vi "Vor Lin Check Benutzerabfrage.vi"() -> ()   [LabVIEW 2020, in "Linearisierung v2.lvlib" / "Gasteiler.lvlib"]
uses:
  Gasteiler.lvlib
  AK-Komm Gasteiler/Aktionen AK Komm.ctl
  AK-Komm Gasteiler/AK Komm Gasteiler.lvlib
  Lin Daten verwalten Aktionen.ctl
  Stufen Tabelle.ctl
  Aktionen FGV Gasteiler Daten.ctl
  AK-Komm Gasteiler/Alter Gasteiler/Aktionen AK Komm_ALT.ctl
  AK-Komm Gasteiler/Alter Gasteiler/Alter Gasteiler.lvlib
  Allgemein/allgemeine Sub-VIs.lvlib
  Sprachverwaltung/Sprachverwaltung.lvlib
  Visualisierungs Elemente/Zahlen-Eingabefeld.ctl
  Horiba/Horiba GDC.lvlib
  Horiba/Aktion Befehl.ctl
  Sprachverwaltung/FGV Aktion Tabelle zerlegen.ctl
  Visualisierungs Elemente/Button.ctl
panel:
  in  "Stufen Tabelle 2":T1
  in  "Abbrechen":T2
  in  "OK":T2
  out "Stufen Tabelle":T1
  out "AGAK":string[](array[string])
  # "Parameter Kontrolle"
  # "Inlet Gas:"
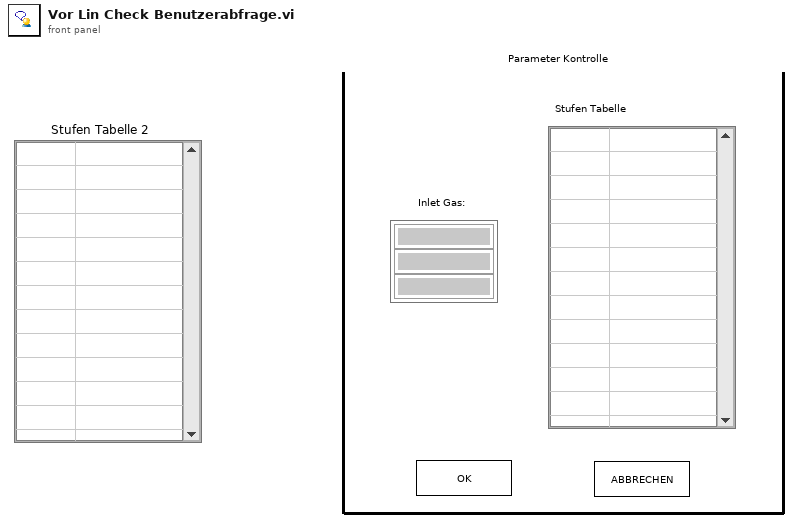
[diagram p1: front panel]
types:
  T1 = typedef "Linearisierung v2.lvlib/Gasteiler.lvlib/Stufen Tabelle.ctl" = string[][]
  T2 = typedef "Button.ctl" = bool
  T3 = typedef "Sprachverwaltung.lvlib/FGV Aktion Tabelle zerlegen.ctl" = enum16{"laden", "vereinzeln", "speichern"}
  T4 = enum8{"Enabled", "Disabled", "Disabled and Grayed Out"}
  T5 = typedef "Linearisierung v2.lvlib/Gasteiler.lvlib/Aktionen FGV Gasteiler Daten.ctl" = enum16{"lesen", "Gasteiler Daten", "Seriellen Param.", "MB-Endwert", "laden", "speichern", "Anforderung", "TCP", "Aufzeichnung Start"}
  T6 = typedef "Linearisierung v2.lvlib/Gasteiler.lvlib/Lin Daten verwalten Aktionen.ctl" = enum16{"lesen", "speichern", "laden", "Lin Daten schr.", "Stufen Tabelle", "Lin Name AK", "Lin Pfad AK", "Umkehren"}
  T7 = typedef "Linearisierung v2.lvlib/Gasteiler.lvlib/AK Komm Gasteiler.lvlib/Aktionen AK Komm.ctl" = enum16{"lesen", "initialisieren", "beenden", "Status", "SMAN", "SREM", "STBY", "ASTF", "ASTZ", "SLST", "AGAT", "EGAK", "AGAK", "AKAK", "ADRU", "SKOP", "SVSA", "SVSZ", "SONO", "SAIR", "SNOX", "ANOX", "SSPL", "SRUC", "SLIN", "ALST", "ETYP", "SVIO", "LCYL", "CCYL", "DCYL", "SCYL", "GCYL", "DRGV", "DRDC"}
  T8 = typedef "Linearisierung v2.lvlib/Gasteiler.lvlib/AK Komm Gasteiler.lvlib/Alter Gasteiler.lvlib/Aktionen AK Komm_ALT.ctl" = enum16{"lesen", "initialisieren", "beenden", "SRES", "STBY", "SREM", "SMAN", "SLIN", "SLCH", "SLST", "SSPL", "AGAT", "ALST", "ASTZ", "ASTF", "AGAK", "EGAK"}
  T9 = typedef "Linearisierung v2.lvlib/Gasteiler.lvlib/Horiba GDC.lvlib/Aktion Befehl.ctl" = enum16{"lesen", "initialisieren", "Beenden", "Standby", "GD/CC", "Info", "Flow", "Alarm", "GD parameter", "GD point", "Durchfluss", "Spuelen1", "Spuelen1 On", "Spuelen1Off", "Spuelen2", "Ventil-Abfrage", "Reset"}
  T10 = typedef "Zahlen-Eingabefeld.ctl" = sgl
  T11 = typedef "Linearisierung v2.lvlib/Gasteiler.lvlib/Gasteiler Daten.ctl" = cluster{"Gasteiler":T12, "Gasteiler Stufen":T13, "Gasteiler Type":T14, "Konfig Gasteiler":T15, "Gasteiler Span Eingänge":u16}
  T12 = typedef "String - Eingabefeld.ctl" = string
  T13 = typedef "Linearisierung v2.lvlib/Gasteiler.lvlib/Gasteiler Stufen.ctl" = u16
  T14 = typedef "Linearisierung v2.lvlib/GasteilerType.ctl" = u16
  T15 = typedef "System Einstellungen V2.lvlib/Gasteiler Auswahl.ctl" = u16
  T16 = typedef "Linearisierung v2.lvlib/Gasteiler.lvlib/Lin Daten.ctl" = cluster{"PrüfgasName":T12, "Verdünnungsgas":T17, "Anzahl Stufen":T10, "Zeitdauer Stufe":T10, "Max Fehler (Sollwert)":T10, "Bearbeiter":T12, "Kalibriergerät":T12, "Mittelwerte":i32, "Komponente":u16, "CalGas Eingang":u16, "Konzentration":sgl}
  T17 = typedef "Linearisierung v2.lvlib/Gasteiler.lvlib/Prüfgas in.ctl" = u16
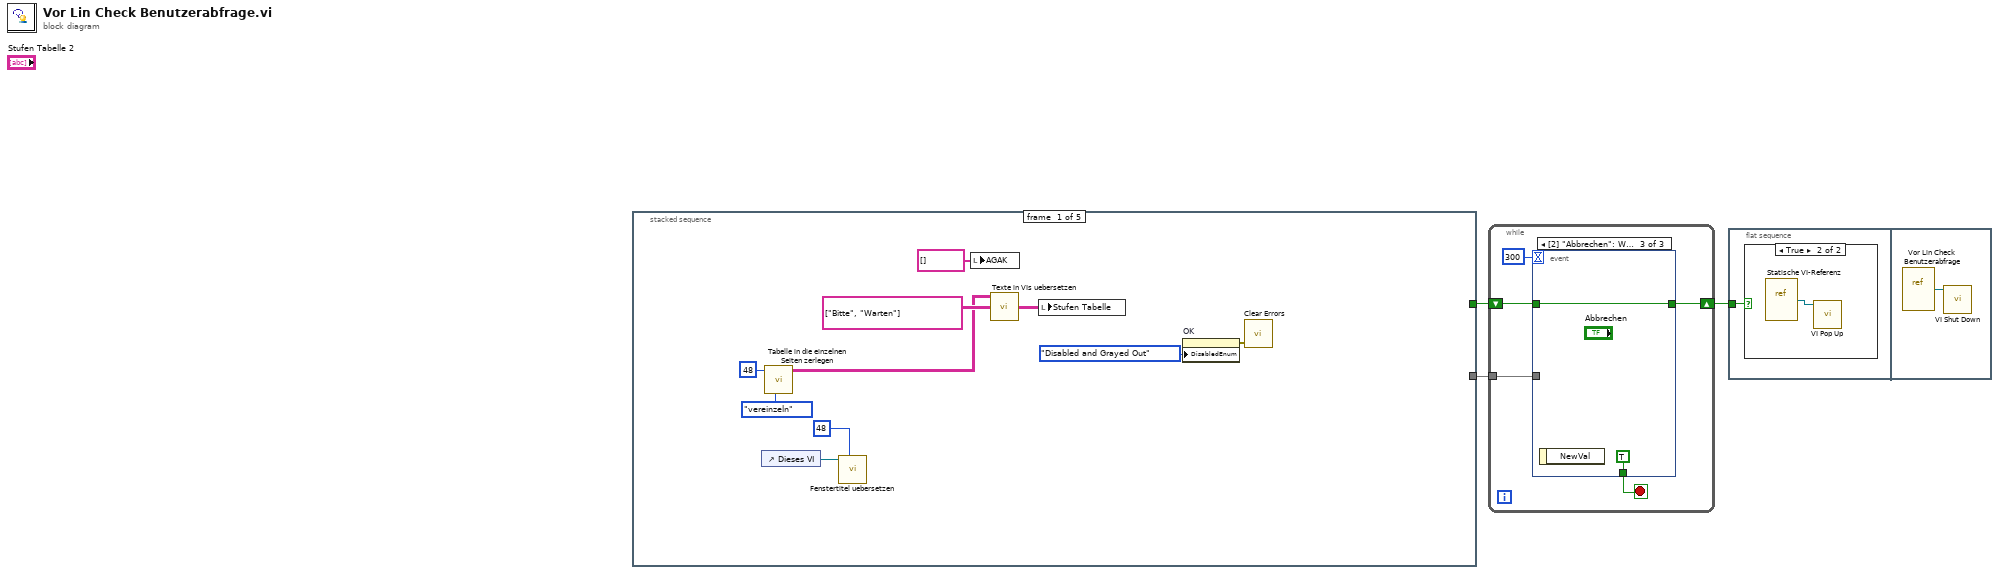
[diagram p0: block diagram]
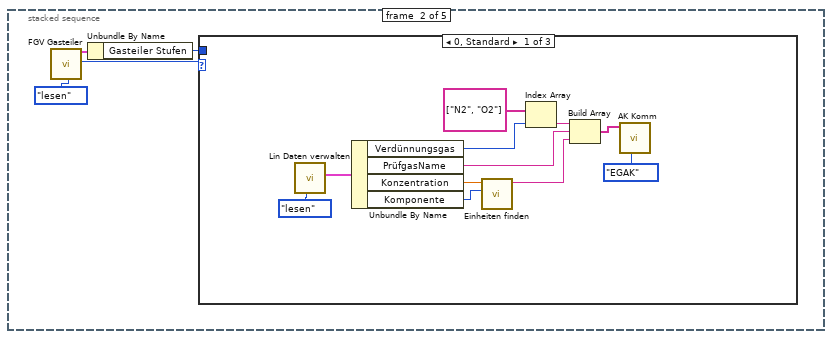
[diagram p3: hidden frame]
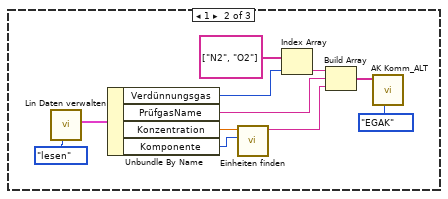
[diagram p4: hidden frame]
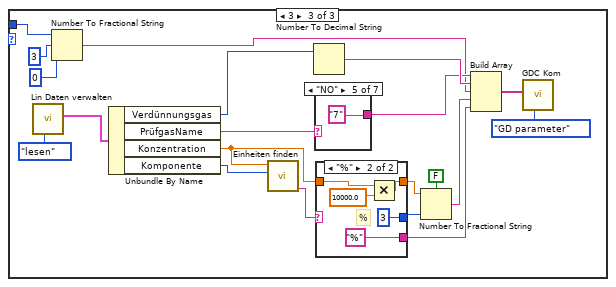
[diagram p5: hidden frame]
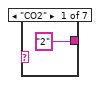
[diagram p6: hidden frame]
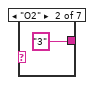
[diagram p7: hidden frame]
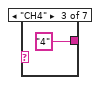
[diagram p8: hidden frame]
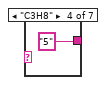
[diagram p9: hidden frame]
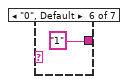
[diagram p10: hidden frame]
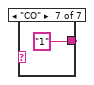
[diagram p11: hidden frame]
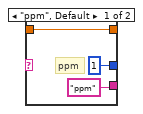
[diagram p12: hidden frame]
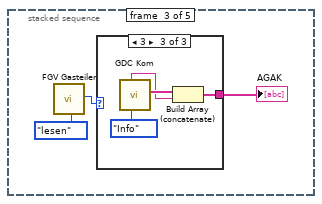
[diagram p13: hidden frame]
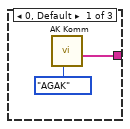
[diagram p14: hidden frame]
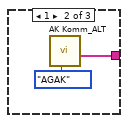
[diagram p15: hidden frame]
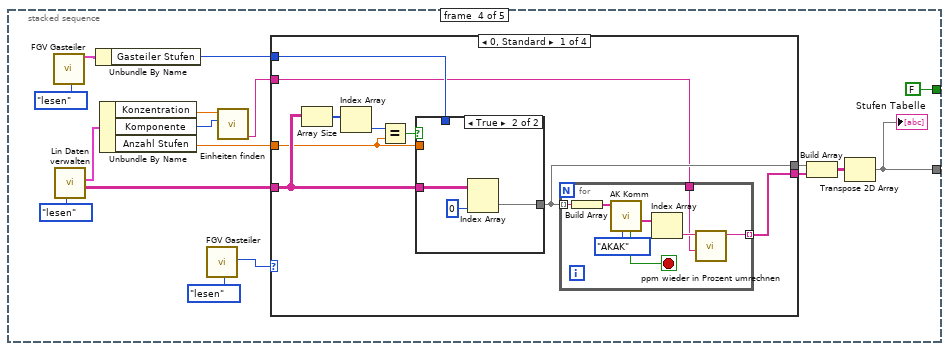
[diagram p16: hidden frame]
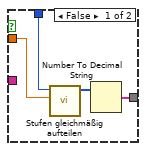
[diagram p17: hidden frame]
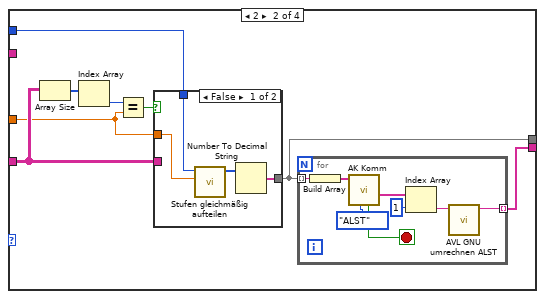
[diagram p18: hidden frame]
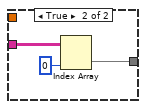
[diagram p19: hidden frame]
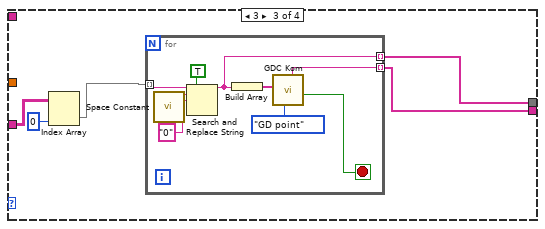
[diagram p20: hidden frame]
diagram:
  n1 = stacked-sequence {
    tunnel: [_ _ _ FALSE _] -> w3
    tunnel: [_ _ _ w99 _] -> w2
    frame #0 {
      n2 = control-ref of="Dieses VI"() -> (w6:refnum<vi>)
      n3 = call "Tabelle in die einzelnen Seiten zerlegen.vi"("Aktion"=FGV_Aktion_Tabelle_zerlegen."vereinzeln", "Index (Seite)"=48) -> ("Sprachliste"=w8:string[][])  [unwired: 7 in, 2 out]
      n4 = call "Fenstertitel uebersetzen.vi"("Index (Seite)"=48, "Dieses VI"=w6) -> ()  [unwired: 8 in, 2 out]
      n5 = local write "AGAK"(string[] [] ("AGAK")) -> ()
      n6 = call "Texte in VIs uebersetzen.vi"("Sprachliste"=w8, "2D String-Array zum Übersetzen"=T1 [["Bitte", "Warten"]] ("Stufen Tabelle")) -> ("2D String-Array zum Übersetzen"=w9:string[][])  [unwired: 9 in, 4 out]
      n7 = local write "Stufen Tabelle"(w9) -> ()
      n8 = property on="OK" class="Bool."("DisabledEnum"=T4."Disabled and Grayed Out" ("Deaktiviert")) -> (error out=w7:errorcluster)  [unwired: 2 in, 1 out]
      n9 = call <vilib>:"Clear Errors.vi"("error in (no error)"=w7) -> ()  [unwired: 5 in, 2 out]
    }
    frame #1 {
      n10 = call "FGV Gasteiler.vi"("Aktionen"=Aktionen_FGV_Gasteiler_Daten."lesen") -> ("Gasteiler Daten"=w15:T11, "Gasteiler Type"=w16:T14)  [unwired: 11 in, 6 out]
      n11 = Unbundle By Name(w15) -> ("Gasteiler Stufen"=w14:T13)
      n12 = case shown="0, Standard" w16 {
        tunnel: w14 -> [_ _ w42]
        frame 0, Default {
          n13 = call "Lin Daten verwalten.vi"("Aktionen"=Lin_Daten_verwalten_Aktionen."lesen") -> ("Lin Daten einzeln"=w23:T16)  [unwired: 5 in, 5 out]
          n14 = Unbundle By Name(w23) -> ("Verdünnungsgas"=w21:T17, "PrüfgasName"=w22:T12, "Konzentration"=w26:sgl, "Komponente"=w27:u16)
          n15 = call "Einheiten finden.vi"("Komponente"=w27, "Wert"=w26) -> ("String"=w25:string)  [unwired: 5 in, 4 out]
          n16 = Index Array(array=string[] ["N2", "O2"] ("Strings []"), index=w21) -> (element=w19:string)
          n17 = Build Array(w19, w22, w25) -> (w18:T12[])
          n18 = call "AK Komm.vi"("Aktionen"=Aktionen_AK_Komm."EGAK", "Daten"=w18) -> ()  [unwired: 3 in, 7 out]
        }
        frame 1 {
          n19 = call "Lin Daten verwalten.vi"("Aktionen"=Lin_Daten_verwalten_Aktionen."lesen") -> ("Lin Daten einzeln"=w34:T16)  [unwired: 5 in, 5 out]
          n20 = Unbundle By Name(w34) -> ("Verdünnungsgas"=w32:T17, "PrüfgasName"=w33:T12, "Konzentration"=w37:sgl, "Komponente"=w38:u16)
          n21 = call "Einheiten finden.vi"("Komponente"=w38, "Wert"=w37) -> ("String"=w36:string)  [unwired: 5 in, 4 out]
          n22 = Index Array(array=string[] ["N2", "O2"] ("Strings []"), index=w32) -> (element=w30:string)
          n23 = Build Array(w30, w33, w36) -> (w29:T12[])
          n24 = call "AK Komm_ALT.vi"("Aktionen_ALT"=Aktionen_AK_Komm_ALT."EGAK", "Daten"=w29) -> ()  [unwired: 5 in, 5 out]
        }
        frame 3 {
          n25 = call "Lin Daten verwalten.vi"("Aktionen"=Lin_Daten_verwalten_Aktionen."lesen") -> ("Lin Daten einzeln"=w58:T16)  [unwired: 5 in, 5 out]
          n26 = Number To Fractional String(number=w42, width (-)=i16 3 ("Breite (-)"), precision (6)=i16 0 ("Genauigkeit (6)")) -> (F-format string=w40:string)  [unwired: 1 in]
          n27 = Unbundle By Name(w58) -> ("Verdünnungsgas"=w53:T17, "PrüfgasName"=w56:T12, "Konzentration"=w55:sgl, "Komponente"=w57:u16)
          n28 = call "Einheiten finden.vi"("Komponente"=w57, "Wert"=w55) -> ("Einheit in String"=w54:string)  [unwired: 5 in, 4 out]
          n29 = Number To Decimal String(number=w53) -> (decimal integer string=w47:string)  [unwired: 1 in]
          n30 = case shown="\"NO\"" w56 {
            tunnel: ["2" "3" "4" "5" "7" "1" "1"] -> w41
            frame "CO2" {
            }
            frame "O2" {
            }
            frame "CH4" {
            }
            frame "C3H8" {
            }
            frame "NO" {
            }
            frame "0", Default {
            }
            frame "CO" {
            }
          }
          n31 = case shown="\"%\"" w54 {
            tunnel: [i16 1 ("Genauigkeit (6)") i16 3 ("Genauigkeit (6)")] -> w51
            tunnel: w55 -> [w68 w73]
            tunnel: [w68 w72] -> w52
            tunnel: ["ppm" "%"] -> w49
            frame "ppm", Default {
              # "ppm"
            }
            frame "%" {
              # "%"
              n32 = Multiply(x=w73, y=T10 10000.0) -> (x*y=w72:T10)
            }
          }
          n33 = Number To Fractional String(use system decimal point (T)=FALSE ("Systemdezimalzeichen verwenden (T)"), number=w52, precision (6)=w51) -> (F-format string=w48:string)  [unwired: 1 in]
          n34 = Build Array(w41, w47, w40, w48, w49) -> (w45:string[])
          n35 = call "GDC Kom.vi"("Befehl"=Aktion_Befehl."GD parameter", "Daten"=w45) -> ()  [unwired: 3 in, 7 out]
        }
      }
    }
    frame #2 {
      n36 = call "FGV Gasteiler.vi"("Aktionen"=Aktionen_FGV_Gasteiler_Daten."lesen") -> ("Gasteiler Type"=w75:T14)  [unwired: 11 in, 7 out]
      n37 = case shown="3" w75 {
        tunnel: [w79 w80 w84] -> w77
        frame 0, Default {
          n38 = call "AK Komm.vi"("Aktionen"=Aktionen_AK_Komm."AGAK") -> ("Empfangsdaten"=w79:string[])  [unwired: 4 in, 6 out]
        }
        frame 1 {
          n39 = call "AK Komm_ALT.vi"("Aktionen_ALT"=Aktionen_AK_Komm_ALT."AGAK") -> ("Empfangsdaten"=w80:string[])  [unwired: 6 in, 4 out]
        }
        frame 3 {
          n40 = call "GDC Kom.vi"("Befehl"=Aktion_Befehl."Info") -> ("Gas"=w83:string[], "Konzentration 2"=w82:string)  [unwired: 4 in, 5 out]
          n41 = Build Array (concatenate)(w83, w82) -> (w84:string[])
        }
      }
      "AGAK" <- w77
    }
    frame #3 {
      n42 = call "FGV Gasteiler.vi"("Aktionen"=Aktionen_FGV_Gasteiler_Daten."lesen") -> ("Gasteiler Daten"=w95:T11)  [unwired: 11 in, 7 out]
      n43 = call "Lin Daten verwalten.vi"("Aktionen"=Lin_Daten_verwalten_Aktionen."lesen") -> ("Stufen Tabelle"=w97:T1, "Lin Daten einzeln"=w90:T16)  [unwired: 5 in, 4 out]
      n44 = Unbundle By Name(w95) -> ("Gasteiler Stufen"=w93:T13)
      n45 = Unbundle By Name(w90) -> ("Konzentration"=w88:sgl, "Komponente"=w87:u16, "Anzahl Stufen"=w96:T10)
      n46 = call "FGV Gasteiler.vi"("Aktionen"=Aktionen_FGV_Gasteiler_Daten."lesen") -> ("Gasteiler Type"=w91:T14)  [unwired: 11 in, 7 out]
      n47 = call "Einheiten finden.vi"("Komponente"=w87, "Wert"=w88) -> ("Einheit in String"=w86:string)  [unwired: 5 in, 4 out]
      n48 = case shown="0, Standard" w91 {
        tunnel: [w111 w134 w151 w164] -> w89
        tunnel: [w110 w133 w150 w165] -> w98
        tunnel: w97 -> [w109 w132 w153 _]
        tunnel: w96 -> [w105 w128 _ w167]
        tunnel: w93 -> [w104 w127 _ w168]
        tunnel: w86 -> [w103 _ _ _]
        frame 0, Default {
          n49 = Array Size(array=w109) -> (size(s)=w108:i32[])
          n50 = Index Array(array=w108) -> (element=w107:i32)  [unwired: 1 in]
          n51 = Equal?(x=w107, y=w105) -> (x = y?=w106:bool)
          n52 = case shown="True" w106 {
            tunnel: [w114 w118] -> w110
            tunnel: w109 -> [_ w116]
            tunnel: w105 -> [w113 _]
            tunnel: w104 -> [w112 _]
            frame False {
              n53 = call "Stufen gleichmäßig aufteilen.vi"("Stufen"=w113, "Anzahl"=w112) -> ("Stufen"=w115:u16[])  [unwired: 9 in]
              n54 = Number To Decimal String(number=w115) -> (decimal integer string=w114:string[])  [unwired: 1 in]
            }
            frame True {
              n55 = Index Array(array=w116, index (col)=0 ("Deaktivierter Index (Spalte)")) -> (element=w118:string[])  [unwired: 1 in]
            }
          }
          n56 = for {
            tunnel: w110 -> [w125] mode=indexing
            tunnel: [w120] -> w111 mode=indexing
            tunnel: w103 -> [w119]
            stop <- w122 stop-if-true
            n57 = Build Array(w125) -> (w124:string[])
            n58 = call "AK Komm.vi"("Aktionen"=Aktionen_AK_Komm."AKAK", "Daten"=w124) -> ("Empfangsdaten"=w123:string[], "Störung Kommunikation"=w122:bool)  [unwired: 3 in, 5 out]
            n59 = Index Array(array=w123) -> (element=w121:string)  [unwired: 1 in]
            n60 = call "ppm wieder in Prozent umrechnen.vi"("Einheit"=w119, "Werteingang"=w121) -> ("Wertausgang"=w120:string)  [unwired: 9 in]
          }
        }
        frame 2 {
          n61 = Array Size(array=w132) -> (size(s)=w131:i32[])
          n62 = Index Array(array=w131) -> (element=w130:i32)  [unwired: 1 in]
          n63 = Equal?(x=w130, y=w128) -> (x = y?=w129:bool)
          n64 = case shown="False" w129 {
            tunnel: [w137 w141] -> w133
            tunnel: w132 -> [_ w139]
            tunnel: w128 -> [w136 _]
            tunnel: w127 -> [w135 _]
            frame False {
              n65 = call "Stufen gleichmäßig aufteilen.vi"("Stufen"=w136, "Anzahl"=w135) -> ("Stufen"=w138:u16[])  [unwired: 9 in]
              n66 = Number To Decimal String(number=w138) -> (decimal integer string=w137:string[])  [unwired: 1 in]
            }
            frame True {
              n67 = Index Array(array=w139, index (col)=0 ("Deaktivierter Index (Spalte)")) -> (element=w141:string[])  [unwired: 1 in]
            }
          }
          n68 = for {
            tunnel: w133 -> [w148] mode=indexing
            tunnel: [w143] -> w134 mode=indexing
            stop <- w145 stop-if-true
            n69 = Build Array(w148) -> (w147:string[])
            n70 = call "AK Komm.vi"("Aktionen"=Aktionen_AK_Komm."ALST", "Daten"=w147) -> ("Empfangsdaten"=w146:string[], "Störung Kommunikation"=w145:bool)  [unwired: 3 in, 5 out]
            n71 = Index Array(array=w146, index=1 ("Index")) -> (element=w144:string)
            n72 = call "AVL GNU umrechnen ALST.vi"("Teilerstufe in%"=w144) -> ("Konzentration"=w143:string)  [unwired: 10 in]
          }
        }
        frame 3 {
          n73 = Index Array(array=w153, index (col)=0 ("Deaktivierter Index (Spalte)")) -> (element=w152:string[])  [unwired: 1 in]
          n74 = for {
            tunnel: w152 -> [w155] mode=indexing
            tunnel: [w160] -> w151 mode=indexing
            tunnel: [w156] -> w150 mode=indexing
            stop <- w161 stop-if-true
            n75 = call <vilib>:"Space Constant.vi"() -> ("String"=w159:string)
            n76 = Search and Replace String(replace all?=TRUE ("Alle ersetzen? (F)"), input string=w155, search string=w159, replace string="0" ("Ersetzungs-String (\"\")")) -> (result string=w156:string)  [unwired: 4 in, 3 out]
            n77 = Build Array(w156) -> (w162:string[])
            n78 = call "GDC Kom.vi"("Befehl"=Aktion_Befehl."GD point", "Daten"=w162) -> ("Status (alarm)"=w161:bool, "Konzentration"=w160:string)  [unwired: 3 in, 5 out]
          }
        }
        frame 1 {
          n79 = local read "AGAK"() -> (w166:string[])
          n80 = call "Stufen gleichmäßig aufteilen.vi"("Stufen"=w167, "Anzahl"=w168) -> ("Stufen"=w171:u16[])  [unwired: 9 in]
          n81 = Number To Decimal String(number=w171) -> (decimal integer string=w165:string[])  [unwired: 1 in]
          n82 = Index Array(array=w166, index=2 ("Index")) -> (element=w174:string)
          n83 = Fract/Exp String To Number(use system decimal point (T)=TRUE ("Systemdezimalzeichen verwenden (T)"), string=w174, default (0 dbl)=sgl 0.0 ("Standard (0 DBL)")) -> (number=w175:sgl)  [unwired: 1 in, 1 out]
          n84 = call "AK Komm_ALT.vi"("Aktionen_ALT"=Aktionen_AK_Komm_ALT."ALST") -> ("Empfangsdaten"=w170:string[])  [unwired: 6 in, 4 out]
          n85 = call "Stufen berechnen.vi"("Empfangsdaten"=w170, "Konzentration"=w175, "Stufen"=w171) -> ("Stufen Tabelle"=w164:string[])  [unwired: 7 in, 1 out]
        }
      }
      n86 = Build Array(w98, w89) -> (w102:string[][])
      n87 = Transpose 2D Array(2D array=w102) -> (transposed array=w99:string[][])
      "Stufen Tabelle" <- w99
    }
    frame #4 {
      n88 = call "FGV Gasteiler.vi"("Aktionen"=Aktionen_FGV_Gasteiler_Daten."lesen") -> ("Gasteiler Type"=w178:T14)  [unwired: 11 in, 7 out]
      n89 = case shown="3" w178 {
        frame 0, Default {
        }
        frame 3 {
          n90 = call "GDC Kom.vi"("Befehl"=Aktion_Befehl."Standby") -> ()  [unwired: 4 in, 7 out]
        }
      }
      n91 = property on="OK" class="Bool."("DisabledEnum"=T4."Enabled" ("Deaktiviert")) -> (error out=w179:errorcluster)  [unwired: 2 in, 1 out]
      n92 = call <vilib>:"Clear Errors.vi"("error in (no error)"=w179) -> ()  [unwired: 5 in, 2 out]
    }
  }
  n93 = while {
    shift-right: [w184] -> w1
    shift-left: w3 -> [w183]
    tunnel: w2 -> [w182]
    stop <- w185 stop-if-true
    n94 = event shown="[2] \"Abbrechen\": Wertänderung" {
      selector: _ -> [_ _ _]
      dyn-events: _ -> [_ _ _]
      timeout: 300 -> [_ _ _]
      tunnel: [_ TRUE TRUE] -> w185
      tunnel: [w187 "OK" w193] -> w184
      tunnel: w183 -> [w187 _ w193]
      tunnel: w182 -> [_ w188 _]
      event Timeout {
        n95 = event-data() -> ()  [unwired: 1 in, 2 out]
      }
      event Value Change {
        n96 = event-data() -> ()  [unwired: 1 in, 1 out]
        n97 = call "Lin Daten verwalten.vi"("Aktionen"=Lin_Daten_verwalten_Aktionen."Stufen Tabelle", "Stufen Tabelle"=w188) -> ()  [unwired: 4 in, 6 out]
      }
      event Value Change {
        n98 = event-data() -> ()  [unwired: 1 in, 1 out]
      }
    }
  }
  n99 = flat-sequence {
    tunnel: w1 -> [w194]
    frame #0 {
      n100 = case shown="True" w194 {
        frame False {
        }
        frame True {
          n101 = vi-ref "Statische VI-Referenz"() -> ("vi reference"=w195:refnum<vi>)
          n102 = call "VI Pop Up.vi"("VI Referenz"=w195) -> ()  [unwired: 11 in]
        }
      }
    }
    frame #1 {
      n103 = vi-ref "Vor Lin Check Benutzerabfrage.vi"() -> (w196:refnum<vi>)
      n104 = call "VI Shut Down.vi"("VI Referenz"=w196) -> ()  [unwired: 11 in]
    }
  }
